vi "PacketsToJSON.vi"(6 "StreamType(Raw)":T1, 8 "ErrorIn":errorcluster, 10 "Packets":T2[](array[typedef]) {"MeasurementConfig"."Resolution[b]" min=4 max=16 step=1; "MeasurementConfig"."Frequency" min=1 max=10000000 step=1}, 11 "JSONIn":refnum<class "JSON Object.lvclass">) -> (0 "ErrorOut":errorcluster, 2 "JSONPacket":string, 3 "JSONOut":refnum<class "JSON Object.lvclass">)   [LabVIEW 2016]
doc: "Convert Packets to JSON"
uses:
  <vilib>/addons/JSON API/JSON Object/JSON Object.lvclass
  D:/Programy/National Instruments/LabVIEW 2016/vi.lib/addons/JSON API/JSON Value/JSON Value.lvclass
  FallSensor/Packet.ctl
  FallSensor/Sample.ctl
  FallSensor/Reading.ctl
  FallSensor/MeasurementConfig.ctl
  FallSensor/Measurement/AccelFSRange.ctl
  FallSensor/Measurement/GyroFSRange.ctl
  JSONStreamType.ctl
  <vilib>/addons/JSON API/JSON Object/Set Object Item by name.vi
  <vilib>/addons/JSON API/JSON Value/Get as JSON string.vi
  <vilib>/addons/JSON API/JSON Array/JSON Array.lvclass
  <vilib>/addons/JSON API/JSON Array/Set JSON Array.vi
  <vilib>/addons/JSON API/JSON Value/Get as JSON string (pretty).vi
  <vilib>/addons/JSON API/JSON Value/Get Item by name array.vi
  <vilib>/addons/JSON API/JSON Value/JSON Value.lvclass
  <vilib>/addons/JSON API/Get Polymorphic/JSON GetSet.lvlib
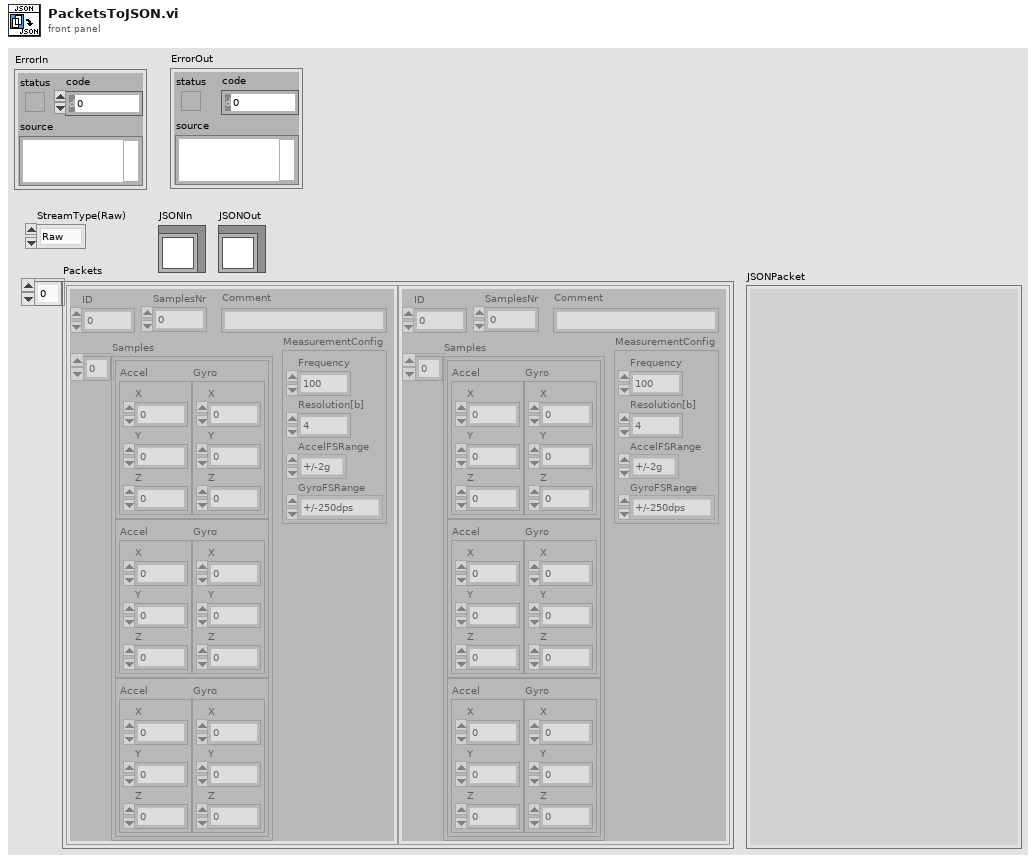
[diagram p1: front panel]
types:
  T1 = typedef "JSONStreamType.ctl" = enum16{"Raw", "Pretty"}
  T2 = typedef "Packet.ctl" = cluster{"ID":u32, "SamplesNr":u32, "Samples":T3[], "MeasurementConfig":T5, "Comment":string}
  T3 = typedef "Sample.ctl" = cluster{"Accel":T4, "Gyro":T4}
  T4 = typedef "Reading.ctl" = cluster{"X":i16, "Y":i16, "Z":i16}
  T5 = typedef "MeasurementConfig.ctl" = cluster{"Frequency":u32, "Resolution[b]":u32, "AccelFSRange":T6, "GyroFSRange":T7}
  T6 = typedef "AccelFSRange.ctl" = enum16{"+/-2g", "+/-4g", "+/-8g", "+/-16g"}
  T7 = typedef "GyroFSRange.ctl" = enum16{"+/-250dps", "+/-500dps", "+/-1000dps", "+/-2000dps"}
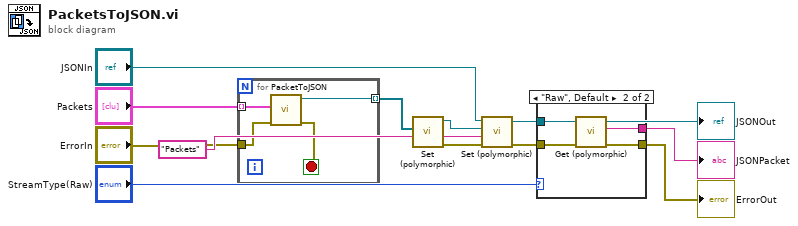
[diagram p0: block diagram]
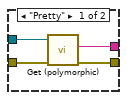
[diagram p2: hidden frame]
diagram:
  n1 = for {
    tunnel: "ErrorIn" -> [w15]
    tunnel: "Packets" -> [w16] mode=indexing
    tunnel: [w13] -> w8 mode=indexing
    stop <- w14 stop-if-true
    n2 = call "PacketToJSON.vi"("ErrorIn"=w15, "Packet"=w16) -> ("ErrorOut"=w14:errorcluster, "JSONOut"=w13:refnum<class "JSON Object.lvclass">)  [unwired: 7 in, 1 out]
  }
  n3 = call-poly <vilib>:"Set (polymorphic).vi"("Array"=w8) -> ("error out"=w11:errorcluster, "JSON Array out"=w12:refnum<class "JSON Array.lvclass">)  [unwired: 9 in]
  n4 = call-poly <vilib>:"Set (polymorphic).vi"("error in (no error)"=w11, "name"="Packets", "Value"=w12, "JSON Object in"="JSONIn") -> ("error out"=w7:errorcluster, "JSON Object out"=w5:refnum<class "JSON Object.lvclass">)  [unwired: 5 in, 1 out]
  "JSONOut" <- w5
  n5 = case shown="\"Raw\", Default" "StreamType(Raw)" {
    tunnel: w7 -> [w20 w24]
    tunnel: [w19 w23] -> w6
    tunnel: w5 -> [w18 w22]
    tunnel: [w17 w21] -> w2
    frame "Pretty" {
      n6 = call-poly <vilib>:"Get (polymorphic).vi"("error in (no error)"=w20, "JSON Value in"=w18) -> ("error out"=w17:errorcluster, "<JSON>"=w19:string)  [unwired: 8 in]
    }
    frame "Raw", Default {
      n7 = call-poly <vilib>:"Get (polymorphic).vi"("error in (no error)"=w24, "JSON Value in"=w22) -> ("error out"=w21:errorcluster, "<JSON>"=w23:string)  [unwired: 8 in]
    }
  }
  "ErrorOut" <- w2
  "JSONPacket" <- w6
